vi "T Vector Predictive Filter.vi"(6 "threshold":dbl=0.0625 format="%#_13g", 9 "Tag ID":i32, 10 "t Translation Vector":dbl[](array[numeric]) format="%#.6f") -> (2 "t Translation Vector Prodictive filtered":dbl[](array[numeric]))   [LabVIEW 2025]
uses:
  Predictive Filter Cluster.ctl
panel:
  out "Predictive Filtered Data":dbl[][](array[numeric])
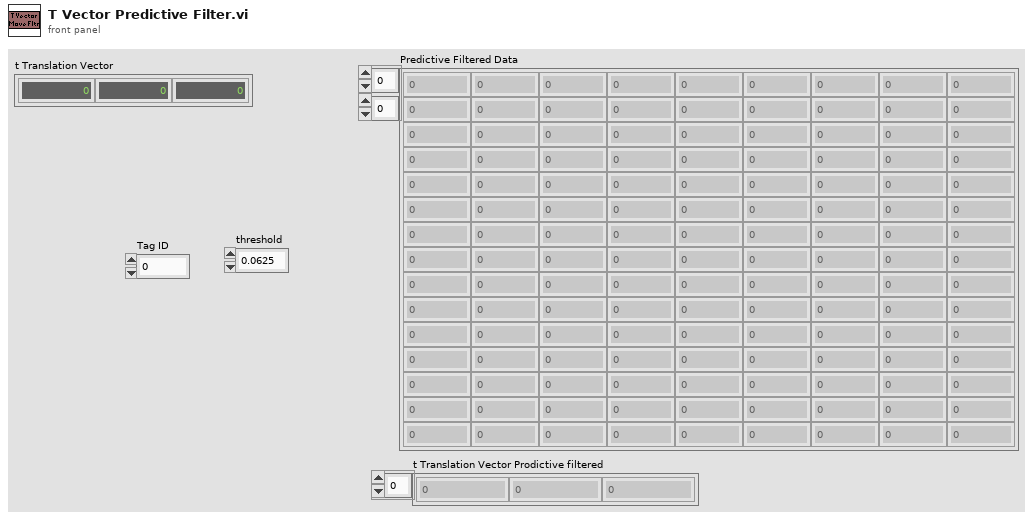
[diagram p1: front panel]
types:
  T1 = typedef "Predictive Filter Cluster.ctl" = cluster{"Previous Position ":dbl[][], "Filter Factor a":dbl[], "Velocity Previous":dbl[][], "Filter Factor ß":dbl[], "Age by tag":u32[]}
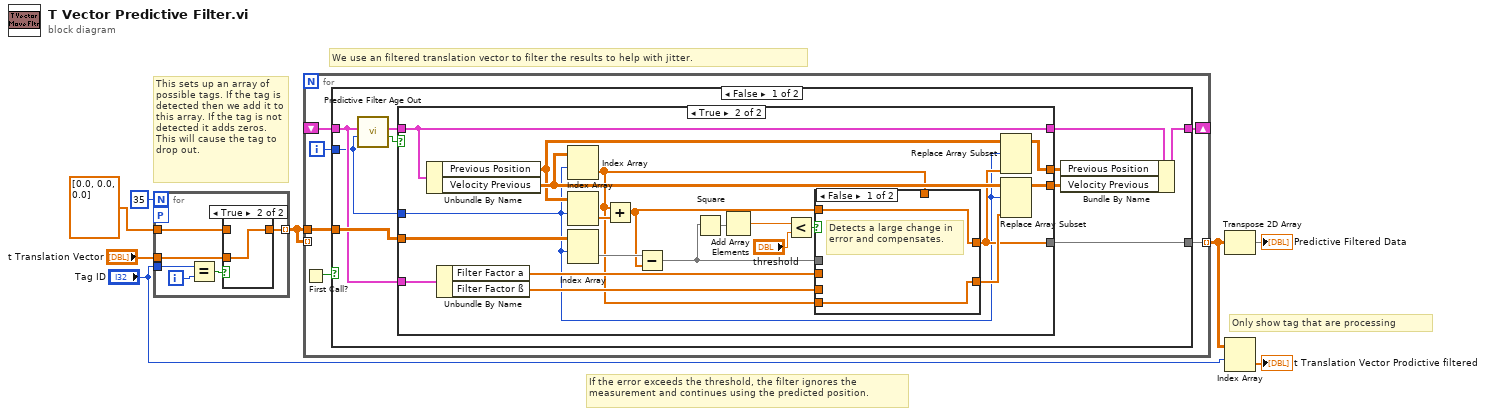
[diagram p0: block diagram]
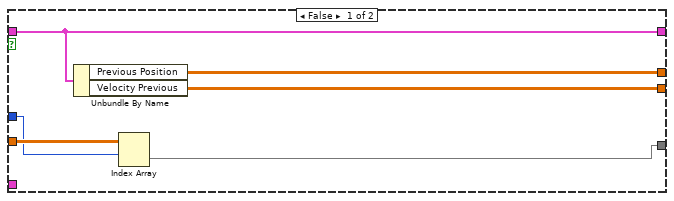
[diagram p2: hidden frame]
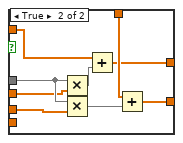
[diagram p3: hidden frame]
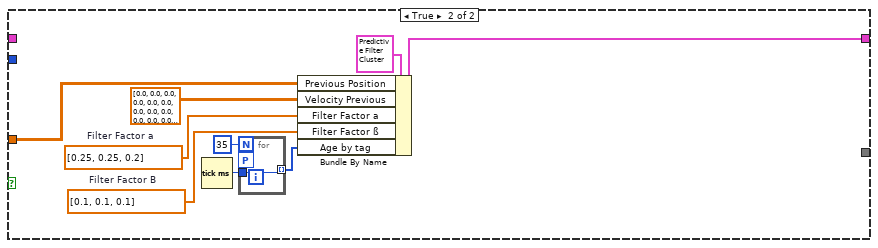
[diagram p4: hidden frame]
diagram:
  # "If the error exceeds the threshold, the filter ignores the measurement and continues using the predicted position."
  # "Only show tag that are processing"
  # "We use an filtered translation vector to filter the results to help with jitter."
  # "This sets up an array of possible tags. If the tag is detected then we add it to this array. If the tag is not detected it adds zeros. This will cause the tag to drop out."
  n1 = for {
    N: 35 -> [_]
    tunnel: dbl[] [0.0, 0.0, 0.0] ("f") -> [w14]
    tunnel: "t Translation Vector" -> [w9]
    tunnel: [w13] -> w5 mode=indexing
    tunnel: "Tag ID" -> [w11]
    workers-P: _ -> [_]
    i -> [w12]
    n2 = Equal?(x=w11, y=w12) -> (x = y?=w10:bool)
    n3 = case shown="True" w10 {
      tunnel: w9 -> [_ w16]
      tunnel: [w15 w16] -> w13
      tunnel: w14 -> [w15 _]
      frame False {
      }
      frame True {
      }
    }
  }
  n4 = for {
    shift-right: [w22] -> _
    shift-left: _ -> [w20]
    tunnel: [w19] -> w2 mode=indexing
    tunnel: w5 -> [w21]
    tunnel: w5 -> [_] mode=indexing
    i -> [w17]
    n5 = First Call?() -> (First Call?: T/F=w18:bool)
    n6 = case shown="False" w18 {
      tunnel: [w32 w78] -> w22
      tunnel: w21 -> [w31 w76]
      tunnel: w20 -> [w26 _]
      tunnel: [w30 _] -> w19
      tunnel: w17 -> [w23 _]
      frame False {
        n7 = call "Predictive Filter Age Out.vi"("Index"=w23, "Predictive Filter Cluster in"=w26) -> ("Process"=w24:bool, "Predictive Filter Cluster out"=w25:T1)  [unwired: 8 in]
        n8 = case shown="True" w24 {
          tunnel: w31 -> [w38 w58]
          tunnel: w26 -> [_ w59]
          tunnel: [w37 w51] -> w30
          tunnel: w25 -> [w36 w57]
          tunnel: [w36 w57] -> w29
          tunnel: [w34 w56] -> w28
          tunnel: [w35 w55] -> w27
          tunnel: w23 -> [w33 w39]
          frame False {
            n9 = Unbundle By Name(w36) -> ("Previous Position"=w35:dbl[][], "Velocity Previous"=w34:dbl[][])
            n10 = Index Array(array=w38, index (row)=w33) -> (element=w37:dbl[])  [unwired: 1 in]
          }
          frame True {
            n11 = Unbundle By Name(w57) -> ("Previous Position"=w47:dbl[][], "Velocity Previous"=w54:dbl[][])
            n12 = Unbundle By Name(w59) -> ("Filter Factor a"=w50:dbl[], "Filter Factor ß"=w49:dbl[])
            n13 = Index Array(array=w54, index (row)=w39) -> (element=w41:dbl[])  [unwired: 1 in]
            n14 = Index Array(array=w47, index (row)=w39) -> (element=w44:dbl[])  [unwired: 1 in]
            n15 = Index Array(array=w58, index (row)=w39) -> (element=w53:dbl[])  [unwired: 1 in]
            n16 = Add(x=w41, y=w44) -> (x+y=w48:dbl[])
            n17 = Subtract(x=w53, y=w48) -> (x-y=w46:dbl[])
            n18 = Square(x=w46) -> (x^2=w45:dbl[])
            n19 = Add Array Elements(numeric array=w45) -> (sum=w40:dbl)
            n20 = Less?(x=w40, y="threshold") -> (x < y?=w42:bool)
            n21 = case shown="False" w42 {
              tunnel: w41 -> [_ w70]
              tunnel: w46 -> [_ w69]
              tunnel: [w61 w67] -> w52
              tunnel: [w60 w66] -> w51
              tunnel: w50 -> [_ w65]
              tunnel: w49 -> [_ w64]
              tunnel: w48 -> [w60 w63]
              tunnel: w41 -> [w61 _]
              frame False {
                # "Detects a large change in error and compensates."
              }
              frame True {
                n22 = Multiply(x=w69, y=w65) -> (x*y=w62:dbl[])
                n23 = Multiply(x=w69, y=w64) -> (x*y=w68:dbl[])
                n24 = Add(x=w63, y=w62) -> (x+y=w66:dbl[])
                n25 = Add(x=w70, y=w68) -> (x+y=w67:dbl[])
              }
            }
            n26 = Replace Array Subset(array=w47, new element=w51, index (row)=w39) -> (w55:dbl[][])  [unwired: 1 in]
            n27 = Replace Array Subset(array=w54, new element=w52, index (row)=w39) -> (w56:dbl[][])  [unwired: 1 in]
          }
        }
        n28 = Bundle By Name(cluster=w29, "Previous Position"=w27, "Velocity Previous"=w28) -> (w32:T1)
      }
      frame True {
        w74 = dbl[] [0.1, 0.1, 0.1]  # Filter Factor B
        w75 = dbl[] [0.25, 0.25, 0.2]  # Filter Factor a
        n29 = Tick Count (ms)() -> (millisecond timer value=w73:u32)
        n30 = for {
          N: 35 -> [_]
          tunnel: w73 -> [w80]
          tunnel: [w80] -> w71 mode=indexing
          workers-P: _ -> [_]
        }
        n31 = Bundle By Name(cluster=T1 {"Previous Position "=[], "Filter Factor a"=[0.25, 0.25, 0.2], "Velocity Previous"=[], "Filter Factor ß"=[0.1, 0.1, 0.1], "Age by tag"=[]}, "Previous Position"=w76, "Velocity Previous"=dbl[][] [[0.0, 0.0, 0.0, 0.0], [0.0, 0.0, 0.0, 0.0], [0.0, 0.0, 0.0, 0.0], [0.0, 0.0, 0.0, 0.0], [0.0, 0.0, 0.0, 0.0], [0.0, 0.0, 0.0, 0.0], [0.0, 0.0, 0.0, 0.0], [0.0, 0.0, 0.0, 0.0], [0.0, 0.0, 0.0, 0.0], [0.0, 0.0, 0.0, 0.0], [0.0, 0.0, 0.0, 0.0], [0.0, 0.0, 0.0, 0.0], [0.0, 0.0, 0.0, 0.0], [0.0, 0.0, 0.0, 0.0], [0.0, 0.0, 0.0, 0.0], [0.0, 0.0, 0.0, 0.0], [0.0, 0.0, 0.0, 0.0], [0.0, 0.0, 0.0, 0.0], [0.0, 0.0, 0.0, 0.0], [0.0, 0.0, 0.0, 0.0], [0.0, 0.0, 0.0, 0.0], [0.0, 0.0, 0.0, 0.0], [0.0, 0.0, 0.0, 0.0], [0.0, 0.0, 0.0, 0.0], [0.0, 0.0, 0.0, 0.0], [0.0, 0.0, 0.0, 0.0], [0.0, 0.0, 0.0, 0.0], [0.0, 0.0, 0.0, 0.0], [0.0, 0.0, 0.0, 0.0], [0.0, 0.0, 0.0, 0.0], [0.0, 0.0, 0.0, 0.0], [0.0, 0.0, 0.0, 0.0], [0.0, 0.0, 0.0, 0.0], [0.0, 0.0, 0.0, 0.0], [0.0, 0.0, 0.0, 0.0], [0.0, 0.0, 0.0, 0.0]], "Filter Factor a"=w75, "Filter Factor ß"=w74, "Age by tag"=w71) -> (w78:T1)
      }
    }
  }
  n32 = Transpose 2D Array(2D array=w2) -> (transposed array=→"Predictive Filtered Data":dbl[][])
  n33 = Index Array(array=w2, index (row)="Tag ID") -> (element=→"t Translation Vector Prodictive filtered":dbl[])  [unwired: 1 in]
